vi "FG RightVelocity.vi"(2 "FG Action (Read)":T1, 3 "Right Velocity In (RPM)":dbl) -> (1 "Right Velocity Out (RPM)":dbl)   [LabVIEW 2009]
uses:
  Actions for FG's.ctl
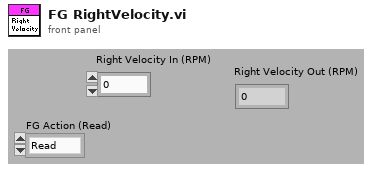
[diagram p1: front panel]
types:
  T1 = typedef "Actions for FG's.ctl" = enum16{"Read", "Write"}
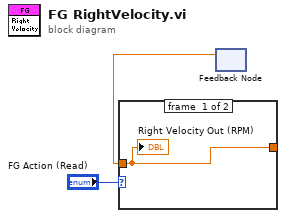
[diagram p0: block diagram]
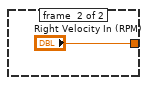
[diagram p2: hidden frame]
diagram:
  n1 = feedback #1() -> (w1:dbl)  [unwired: 1 in]
  n2 = case shown="\"Write\"" "FG Action (Read)" {
    tunnel: [w4 "Right Velocity In (RPM)"] -> w2
    tunnel: w1 -> [w4 _]
    frame #0 {
      "Right Velocity Out (RPM)" <- w4
    }
    frame #1 {
    }
  }
